vi "niRFUtil RFHS FIFO Get Status.vi"(0 "Fifo ID":T1, 11 "error in (no error)":errorcluster) -> (4 "Fifo ID (out)":T1, 6 "size":u32, 8 "capacity":u32, 15 "error out":errorcluster)   [LabVIEW 2015, in "niRFUtil.lvlib"]
uses:
  niRFUtil.lvlib
  niRFUtil RFHS FIFO Reference.ctl
  niRFUtil RFHS FIFO.ctl
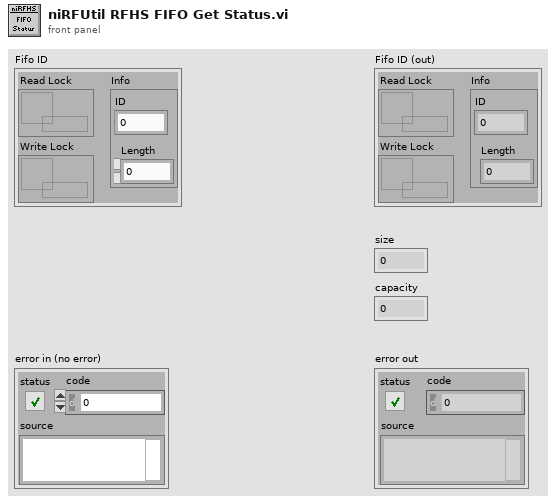
[diagram p1: front panel]
types:
  T1 = typedef "niRFUtil.lvlib/niRFUtil RFHS FIFO Reference.ctl" = cluster{"Read Lock":refnum<data-value>, "Info":T2, "Write Lock":refnum<data-value>}
  T2 = typedef "niRFUtil.lvlib/niRFUtil RFHS FIFO.ctl" = cluster{"ID":u64, "Length":u32}
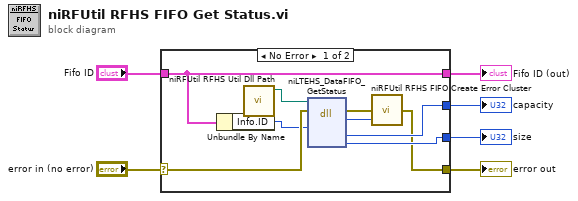
[diagram p0: block diagram]
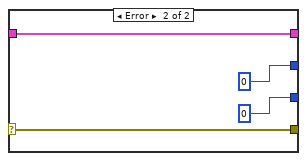
[diagram p2: hidden frame]
diagram:
  n1 = case shown="No Error" "error in (no error)" {
    selector: "error in (no error)" -> [w15 w19]
    tunnel: [w7 w19] -> w5
    tunnel: "Fifo ID" -> [w10 w18]
    tunnel: [w10 w18] -> w3
    tunnel: [w13 u32 0 ("capacity")] -> w2
    tunnel: [w12 u32 0 ("size")] -> w1
    frame No Error {
      n2 = Unbundle By Name(w10) -> ("Info.ID"=w14:u64)
      n3 = call "niRFUtil RFHS Util Dll Path.vi"() -> ("Path"=w11:path)  [unwired: 7 in, 4 out]
      n4 = dll-call lib="M:/RfProtocols/RFmx/DLLs/niRFHS/trunk/2.0/dist/win32U/niRFHS_generic.dll" fn="niLTEHS_DataFIFO_GetStatus"(path in=w11, error in=w15, "fifoID"=w14) -> (error out=w9:errorcluster, "return type"=w8:i32, "capacity"=w13:u32, "size"=w12:u32)  [unwired: 4 in, 1 out]
      n5 = call "niRFUtil RFHS FIFO Create Error Cluster.vi"("error in (no error)"=w9, "fifo return value"=w8) -> ("error  out"=w7:errorcluster)  [unwired: 12 in, 1 out]
    }
    frame Error {
    }
  }
  "error out" <- w5
  "Fifo ID (out)" <- w3
  "capacity" <- w2
  "size" <- w1
